vi "Main.vi"(11 "Module Admin":refnum<class "Delacor_lib_QMH_Cloneable Module Admin.lvclass">) -> ()   [LabVIEW 2020, in "FGen.lvlib"]
doc: "This template is based off of the Queued Message Handler design pattern and the Queued Message Handler project template that ships with LabVIEW.\n\nThe main difference is that the queue is private to this module and communication between modules is performed via Broadcast and Request events.\n\nRequest events are wrapped in public API methods and are handled in the Event Handling Loop (EHL) of this VI. Any module can register for Broadcast events sent by this module. The EHL generates messages based on user interface actions.\n\nThe Message Handling Loop (MHL) processes messages generated by the EHL, or by other messages. The messages are string values, so new messages can be added easily to the Message Cases case structure in the MHL. Each message cluster can also provide an optional value for Message Data, which is a variant that can be converted to whatever message-specific data is required.\n_____\nBased on DQMH Project Template 6.0.0.91."
uses:
  FGen.lvlib
  <vilib>/Delacor/Delacor QMH/Libraries/Cloneable Module Admin_class/Delacor_lib_QMH_Cloneable Module Admin.lvclass
  C:/Program Files (x86)/National Instruments/LabVIEW 2020/vi.lib/Delacor/Delacor QMH/Libraries/Module Admin_class/Delacor_lib_QMH_Module Admin.lvclass
  Module Data--cluster.ctl
  Generador/Generador.lvclass
  <vilib>/Delacor/Delacor QMH/Libraries/Message Queue_class/Delacor_lib_QMH_Message Queue.lvclass/Delacor_lib_QMH_Message Queue.ctl
  <vilib>/Delacor/Delacor QMH/Libraries/Cloneable Module Admin_class/Delacor_lib_QMH_Cloneable Module Admin.lvclass/Delacor_lib_QMH_Cloneable Module Admin.ctl
  Stop Argument--cluster.ctl
  <vilib>/Delacor/Delacor QMH/Libraries/Module Admin_class/Delacor_lib_QMH_Module Admin.lvclass/Delacor_lib_QMH_Module Admin.ctl
  Set Signal Type Argument--cluster.ctl
  Set to Default Argument--cluster.ctl
  Generate Signal Argument--cluster.ctl
  Generate Signal (Reply Payload)--cluster.ctl
  <vilib>/Utility/miscctls.llb/LVPointTypeDef.ctl
  Generador/Generador.lvclass/Generador.ctl
  <vilib>/Delacor/Delacor QMH/Libraries/Message Queue_class/Delacor_lib_QMH_Enqueue Message (Single).vi
  <vilib>/Delacor/Delacor QMH/Libraries/Cloneable Module Admin_class/Delacor_lib_QMH_Get Module ID.vi
  <vilib>/Delacor/Delacor QMH/Libraries/Module Admin_class/Delacor_lib_QMH_Get External Launch.vi
  <vilib>/Utility/error.llb/Error Cluster From Error Code.vi
  <vilib>/ErrorRing/Error Ring.xnode
  <vilib>/Delacor/Delacor QMH/Libraries/Message Queue_class/Delacor_lib_QMH_Message Queue.lvclass
panel:
  out "error out":errorcluster
  out "Status":string
  in  "Simulate EHL Error":bool
  in  "Simulate MHL Error":bool
  # "Other QMH Modules communicate with this Module via its Public API (wrappers for its Request Events).\n\nThis Module communicates with other Modules via its Broadcast Events.\nAny module that wants to get these messages, just registers for this module's Broadcast events."
  # "This template is for the Delacor Modified Queued Message Handler design pattern.\n\nSee the block diagram for more information on how to use this template."
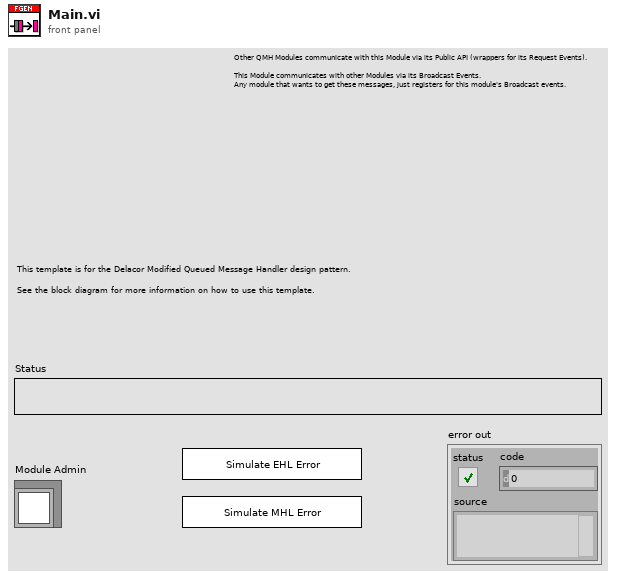
[diagram p1: front panel]
types:
  T1 = typedef "FGen.lvlib/Request Events--cluster.ctl" = cluster{"Stop Module":refnum<user-event>, "Show Panel":refnum<user-event>, "Hide Panel":refnum<user-event>, "Show Diagram":refnum<user-event>, "Get Module Execution Status":refnum<user-event>, "Set Signal Type":refnum<user-event>, "Set to Default":refnum<user-event>, "Generate Signal":refnum<user-event>}
  T2 = typedef "FGen.lvlib/Module Data--cluster.ctl" = cluster{"Status":string, "Generator":refnum<class "Generador.lvclass">}
  T3 = enum32{"invalid lock state", "Not Locked", "Locked (No Password)", "Password-protected"}
  T4 = typedef "FGen.lvlib/Stop Argument--cluster.ctl" = cluster{"Module ID":i32, "Origin":string, "Exit via Stop Module Req?":bool, "Wait for Module to stop?":bool}
  T5 = typedef "FGen.lvlib/Set Signal Type Argument--cluster.ctl" = cluster{"Module ID":i32, "signal type":enum16{"Sine Wave", "Triangle Wave", "Square Wave", "Sawtooth Wave"}}
  T6 = typedef "FGen.lvlib/Set to Default Argument--cluster.ctl" = cluster{"Module ID":i32, "Boolean":bool}
  T7 = typedef "FGen.lvlib/Generate Signal Argument--cluster.ctl" = cluster{"Module ID":i32, "Wait Notifier":refnum<notifier>, "wait for reply":bool}
  T8 = typedef "LVPointTypeDef.ctl" = cluster{"Horizontal":i16, "Vertical":i16}
  T9 = enum32{"Invalid", "Standard", "Closed", "Hidden", "Minimized", "Maximized"}
  T10 = typedef "FGen.lvlib/Generate Signal (Reply Payload)--cluster.ctl" = cluster{"signal out":waveform(dbl), "Generate Signal_error":errorcluster}
  T11 = enum16{"Sine Wave", "Triangle Wave", "Square Wave", "Sawtooth Wave"}
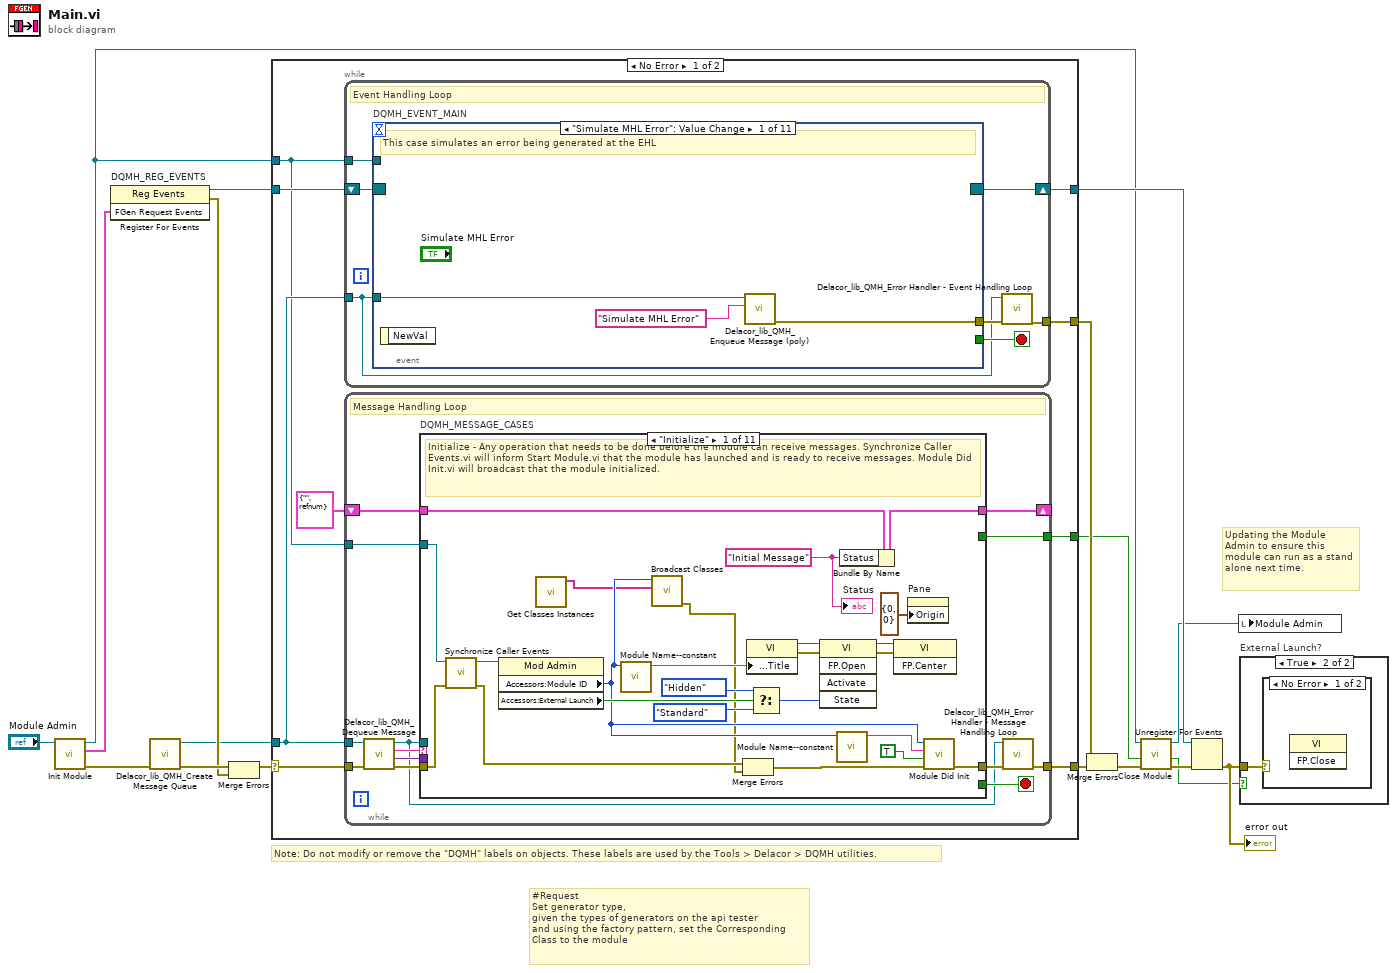
[diagram p0: block diagram]
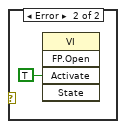
[diagram p3: hidden frame]
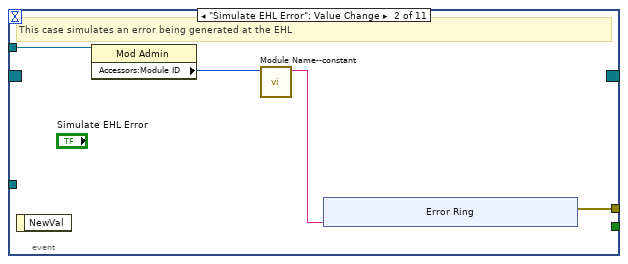
[diagram p4: hidden frame]
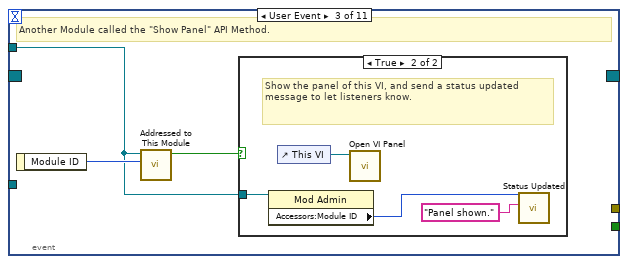
[diagram p5: hidden frame]
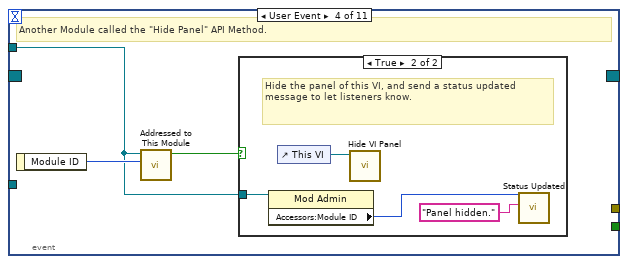
[diagram p7: hidden frame]
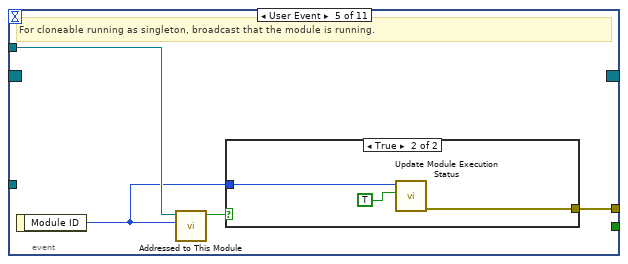
[diagram p9: hidden frame]
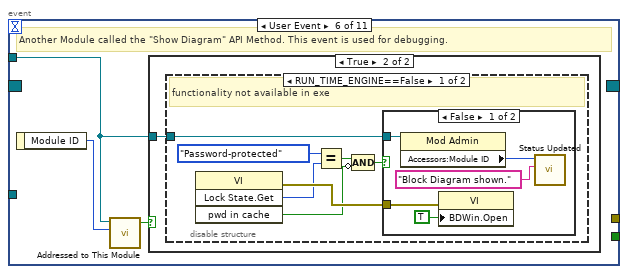
[diagram p11: hidden frame]
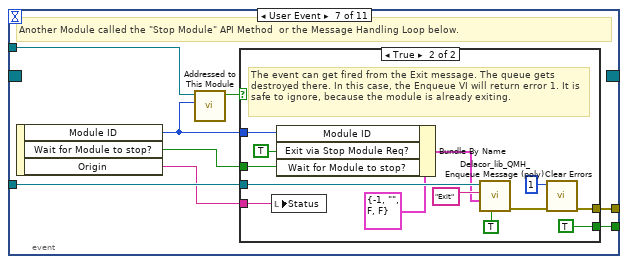
[diagram p15: hidden frame]
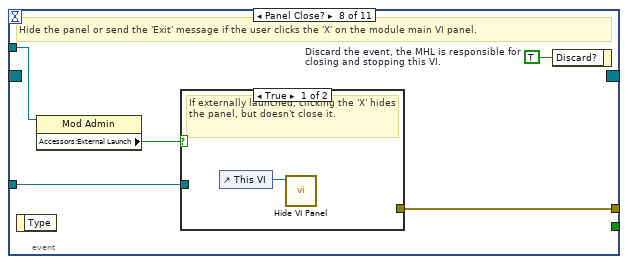
[diagram p17: hidden frame]
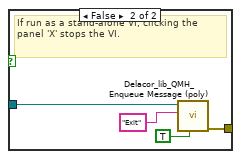
[diagram p18: hidden frame]
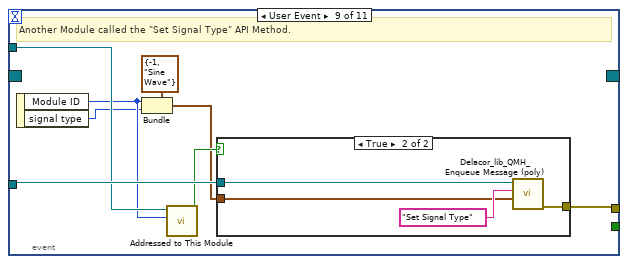
[diagram p19: hidden frame]
diagram:
  # "#Request\nSet generator type, \ngiven the types of generators on the api tester\nand using the factory pattern, set the Corresponding\nClass to the module"
  # "Note: Do not modify or remove the \"DQMH\" labels on objects. These labels are used by the Tools > Delacor > DQMH utilities."
  # "Updating the Module Admin to ensure this module can run as a stand alone next time."
  n1 = call "Init Module.vi"("Cloneable Module Admin in"="Module Admin") -> ("error out"=w15:errorcluster, "FGen Request Events"=w7:T1, "Cloneable Module Admin out"=w4:refnum<class "Delacor_lib_QMH_Cloneable Module Admin.lvclass">)  [unwired: 8 in]
  n2 = register-events "DQMH_REG_EVENTS"(w7) -> (reference out=w8:refnum<event-registration>, error out=w10:errorcluster)  [unwired: 2 in]
  n3 = call <vilib>:"Delacor_lib_QMH_Create Message Queue.vi"("error in"=w15) -> ("error out"=w12:errorcluster, "Message Queue"=w6:refnum<class "Delacor_lib_QMH_Message Queue.lvclass">)  [unwired: 9 in]
  n4 = Merge Errors(w12, w10) -> (w11:errorcluster)
  n5 = case shown="No Error" w11 {
    selector: w11 -> [w25 w304]
    tunnel: [w27 w303] -> w16
    tunnel: [w24 w311] -> w9
    tunnel: w8 -> [w22 w311]
    tunnel: w6 -> [w21 w302]
    tunnel: [w26 _] -> w17
    tunnel: w4 -> [w20 w307]
    tunnel: [w19 _] -> w2
    frame No Error {
      n6 = while {
        tunnel: w21 -> [w28]
        shift-right: [w31] -> w24
        shift-left: w22 -> [w32]
        tunnel: [w33] -> w26
        tunnel: w20 -> [w29]
        stop <- w30 stop-if-true
        # "Event Handling Loop"
        n7 = event "DQMH_EVENT_MAIN" shown="[0] \"Simulate MHL Error\": Value Change" {
          selector: w32 -> [_ _ _ _ _ _ _ _ _ _ _]
          dyn-events: [_ _ _ _ _ _ _ _ _ _ _] -> w31
          timeout: _ -> [_ _ _ _ _ _ _ _ _ _ _]
          tunnel: [_ _ _ _ _ _ w89 _ _ _ _] -> w30
          tunnel: w28 -> [w36 _ _ _ _ _ w92 w108 w124 w136 w149]
          tunnel: [w37 w41 _ _ w66 _ w93 w111 w117 w129 w141] -> w34
          tunnel: w29 -> [_ w40 w49 w56 w64 w70 w91 w109 w122 w134 w147]
          event "Simulate MHL Error": Value Change {
            # "This case simulates an error being generated at the EHL"
            n8 = event-data() -> ()  [unwired: 1 in, 1 out]
            n9 = call-poly <vilib>:"Delacor_lib_QMH_Enqueue Message (poly).vi"("Message"="Simulate MHL Error", "Message Queue in"=w36) -> ("error out"=w37:errorcluster)  [unwired: 8 in, 1 out]
          }
          event "Simulate EHL Error": Value Change {
            # "This case simulates an error being generated at the EHL"
            n10 = event-data() -> ()  [unwired: 1 in, 1 out]
            n11 = property class="Mod Admin"(reference=w40) -> ("Accessors:Module ID"=w39:i32)  [unwired: 1 in, 2 out]
            n12 = call "Module Name--constant.vi"("Module ID"=w39) -> ("Module Name"=w38:string)  [unwired: 10 in]
            n13 = xnode "Error Ring"("parameter 0"=w38) -> ("error out"=w41:errorcluster)
          }
          event User Event {
            # "Another Module called the \"Show Panel\" API Method."
            n14 = event-data() -> ("Module ID"=w50:i32)  [unwired: 1 in]
            n15 = call "Addressed to This Module.vi"("Module ID from Argument"=w50, "Module Admin"=w49) -> ("Addressed to this instance?"=w51:bool)  [unwired: 8 in, 1 out]
            n16 = case shown="True" w51 {
              tunnel: w49 -> [_ w53]
              frame False {
              }
              frame True {
                # "Show the panel of this VI, and send a status updated message to let listeners know."
                n17 = property class="Mod Admin"(reference=w53) -> ("Accessors:Module ID"=w52:i32)  [unwired: 1 in, 2 out]
                n18 = control-ref of="This VI"() -> (w55:refnum<vi>)
                n19 = call "Open VI Panel.vi"("VI"=w55) -> ()  [unwired: 10 in, 1 out]
                n20 = call "Status Updated.vi"("Status"="Panel shown." ("format string"), "Module ID"=w52) -> ()  [unwired: 9 in, 1 out]
              }
            }
          }
          event User Event {
            # "Another Module called the \"Hide Panel\" API Method."
            n21 = event-data() -> ("Module ID"=w57:i32)  [unwired: 1 in]
            n22 = call "Addressed to This Module.vi"("Module ID from Argument"=w57, "Module Admin"=w56) -> ("Addressed to this instance?"=w58:bool)  [unwired: 8 in, 1 out]
            n23 = case shown="True" w58 {
              tunnel: w56 -> [_ w60]
              frame False {
              }
              frame True {
                # "Hide the panel of this VI, and send a status updated message to let listeners know."
                n24 = property class="Mod Admin"(reference=w60) -> ("Accessors:Module ID"=w59:i32)  [unwired: 1 in, 2 out]
                n25 = control-ref of="This VI"() -> (w62:refnum<vi>)
                n26 = call "Hide VI Panel.vi"("VI"=w62) -> ()  [unwired: 10 in, 1 out]
                n27 = call "Status Updated.vi"("Status"="Panel hidden." ("format string"), "Module ID"=w59) -> ()  [unwired: 9 in, 1 out]
              }
            }
          }
          event User Event {
            # "For cloneable running as singleton, broadcast that the module is running."
            n28 = event-data() -> ("Module ID"=w63:i32)  [unwired: 1 in]
            n29 = call "Addressed to This Module.vi"("Module ID from Argument"=w63, "Module Admin"=w64) -> ("Addressed to this instance?"=w65:bool)  [unwired: 8 in, 1 out]
            n30 = case shown="True" w65 {
              tunnel: [_ w69] -> w66
              tunnel: w63 -> [_ w68]
              frame False {
              }
              frame True {
                n31 = call "Update Module Execution Status.vi"("Running?"=TRUE, "Module ID"=w68) -> ("error out"=w69:errorcluster)  [unwired: 9 in]
              }
            }
          }
          event User Event {
            # "Another Module called the \"Show Diagram\" API Method. This event is used for debugging."
            n32 = event-data() -> ("Module ID"=w71:i32)  [unwired: 1 in]
            n33 = call "Addressed to This Module.vi"("Module ID from Argument"=w71, "Module Admin"=w70) -> ("Addressed to this instance?"=w72:bool)  [unwired: 8 in, 1 out]
            n34 = case shown="True" w72 {
              tunnel: w70 -> [_ w73]
              frame False {
              }
              frame True {
                n35 = disable-structure shown="RUN_TIME_ENGINE==False" {
                  disable-tunnel: w73 -> [w74 _]
                  frame condition #0 (active) {
                    # "functionality not available in exe"
                    n36 = invoke class="VI" method="Lock State.Get"() -> (error out=w80:errorcluster, "Get Lock State"=w79:T3, "pwd in cache"=w76:bool)  [unwired: 4 in, 1 out]
                    n37 = Equal?(x=T3."Password-protected", y=w79) -> (x = y?=w77:bool)
                    n38 = Compound Arithmetic op=AND(w77, invert w76) -> (w75:bool)
                    n39 = case shown="False" w75 {
                      tunnel: w80 -> [w85 _]
                      tunnel: w74 -> [w82 _]
                      frame False {
                        n40 = property class="Mod Admin"(reference=w82) -> ("Accessors:Module ID"=w81:i32)  [unwired: 1 in, 2 out]
                        n41 = property class="VI"(error in=w85, "BDWin.Open"=TRUE ("Block Diagram Window:Open")) -> ()  [unwired: 1 in, 2 out]
                        n42 = call "Status Updated.vi"("Status"="Block Diagram shown." ("format string"), "Module ID"=w81) -> ()  [unwired: 9 in, 1 out]
                      }
                      frame True {
                        # "Password-protected VI, and the password is not in the cache. Do not show the diagram."
                      }
                    }
                  }
                  frame condition #1 {
                  }
                }
              }
            }
          }
          event User Event {
            # "Another Module called the \"Stop Module\" API Method  or the Message Handling Loop below."
            n43 = event-data() -> ("Module ID"=w87:i32, "Wait for Module to stop?"=w88:bool, "Origin"=w86:string)  [unwired: 1 in]
            n44 = call "Addressed to This Module.vi"("Module ID from Argument"=w87, "Module Admin"=w91) -> ("Addressed to this instance?"=w90:bool)  [unwired: 8 in, 1 out]
            n45 = case shown="True" w90 {
              tunnel: [_ w105] -> w93
              tunnel: w92 -> [_ w101]
              tunnel: [_ TRUE] -> w89
              tunnel: w88 -> [_ w96]
              tunnel: w87 -> [_ w98]
              tunnel: w86 -> [_ w94]
              frame False {
              }
              frame True {
                # "The event can get fired from the Exit message. The queue gets destroyed there. In this case, the Enqueue VI will return error 1. It is safe to ignore, because the module is already exiting."
                n46 = local write "Status"(w94) -> ()
                n47 = Bundle By Name(cluster=T4 {"Module ID"=-1, "Origin"="", "Exit via Stop Module Req?"=FALSE, "Wait for Module to stop?"=FALSE} ("Stop Argument"), "Module ID"=w98, "Exit via Stop Module Req?"=TRUE, "Wait for Module to stop?"=w96) -> (w95:T4)
                n48 = call-poly <vilib>:"Delacor_lib_QMH_Enqueue Message (poly).vi"("Priority Message? (F)"=TRUE, "Message Data"=w95, "Message"="Exit", "Message Queue in"=w101) -> ("error out"=w106:errorcluster)  [unwired: 6 in, 1 out]
                n49 = call <vilib>:"Clear Errors.vi"("error in (no error)"=w106, "specific error code to clear (0: all)"=1) -> ("error out"=w105:errorcluster)  [unwired: 4 in, 1 out]
              }
            }
          }
          event Panel Close? {
            w110 = TRUE  # Discard the event, the MHL is responsible for closing and stopping this VI.
            # "Hide the panel or send the 'Exit' message if the user clicks the 'X' on the module main VI panel."
            n50 = event-data() -> ()  [unwired: 1 in, 1 out]
            n51 = property class="Mod Admin"(reference=w109) -> ("Accessors:External Launch"=w107:bool)  [unwired: 1 in, 2 out]
            n52 = case shown="True" w107 {
              tunnel: w108 -> [_ w115]
              tunnel: [_ w116] -> w111
              frame True {
                # "If externally launched, clicking the 'X' hides the panel, but doesn't close it."
                n53 = control-ref of="This VI"() -> (w112:refnum<vi>)
                n54 = call "Hide VI Panel.vi"("VI"=w112) -> ()  [unwired: 10 in, 1 out]
              }
              frame False {
                # "If run as a stand-alone VI, clicking the panel 'X' stops the VI."
                n55 = call-poly <vilib>:"Delacor_lib_QMH_Enqueue Message (poly).vi"("Priority Message? (F)"=TRUE, "Message"="Exit", "Message Queue in"=w115) -> ("error out"=w116:errorcluster)  [unwired: 7 in, 1 out]
              }
            }
            n56 = event-data("Discard?"=w110) -> ()  [unwired: 1 in, 1 out]
          }
          event User Event {
            # "Another Module called the \"Set Signal Type\" API Method."
            n57 = event-data() -> ("Module ID"=w119:i32, "signal type"=w118:T11)  [unwired: 1 in]
            n58 = Bundle(cluster=T5 {"Module ID"=-1, "signal type"=enum."Sine Wave"} ("Set Signal Type Argument"), "Module ID"=w119, "signal type"=w118) -> (w120:T5)
            n59 = call "Addressed to This Module.vi"("Module ID from Argument"=w119, "Module Admin"=w122) -> ("Addressed to this instance?"=w123:bool)  [unwired: 8 in, 1 out]
            n60 = case shown="True" w123 {
              tunnel: w124 -> [_ w128]
              tunnel: w120 -> [_ w126]
              tunnel: [_ w125] -> w117
              frame False {
              }
              frame True {
                n61 = call-poly <vilib>:"Delacor_lib_QMH_Enqueue Message (poly).vi"("Message Data"=w126, "Message"="Set Signal Type", "Message Queue in"=w128) -> ("error out"=w125:errorcluster)  [unwired: 7 in, 1 out]
              }
            }
          }
          event User Event {
            # "Another Module called the \"Set to Default\" API Method."
            n62 = event-data() -> ("Module ID"=w131:i32, "Boolean"=w130:bool)  [unwired: 1 in]
            n63 = Bundle(cluster=T6 {"Module ID"=-1, "Boolean"=FALSE} ("Set to Default Argument"), "Module ID"=w131, "Boolean"=w130) -> (w132:T6)
            n64 = call "Addressed to This Module.vi"("Module ID from Argument"=w131, "Module Admin"=w134) -> ("Addressed to this instance?"=w135:bool)  [unwired: 8 in, 1 out]
            n65 = case shown="True" w135 {
              tunnel: w136 -> [_ w140]
              tunnel: w132 -> [_ w138]
              tunnel: [_ w137] -> w129
              frame False {
              }
              frame True {
                n66 = call-poly <vilib>:"Delacor_lib_QMH_Enqueue Message (poly).vi"("Message Data"=w138, "Message"="Set to Default", "Message Queue in"=w140) -> ("error out"=w137:errorcluster)  [unwired: 7 in, 1 out]
              }
            }
          }
          event User Event {
            # "Another Module called the \"Generate Signal\" API Method."
            n67 = event-data() -> ("Module ID"=w144:i32, "Wait Notifier"=w143:refnum<notifier>, "wait for reply"=w142:bool)  [unwired: 1 in]
            n68 = Bundle(cluster=T7 {"Module ID"=-1, "Wait Notifier"=refnum, "wait for reply"=FALSE} ("Generate Signal Argument"), "Module ID"=w144, "Wait Notifier"=w143, "wait for reply"=w142) -> (w145:T7)
            n69 = call "Addressed to This Module.vi"("Module ID from Argument"=w144, "Module Admin"=w147) -> ("Addressed to this instance?"=w148:bool)  [unwired: 8 in, 1 out]
            n70 = case shown="True" w148 {
              tunnel: w149 -> [_ w153]
              tunnel: w145 -> [_ w151]
              tunnel: [_ w150] -> w141
              frame False {
              }
              frame True {
                n71 = call-poly <vilib>:"Delacor_lib_QMH_Enqueue Message (poly).vi"("Message Data"=w151, "Message"="Generate Signal", "Message Queue in"=w153) -> ("error out"=w150:errorcluster)  [unwired: 7 in, 1 out]
              }
            }
          }
        }
        n72 = call-dynamic "Delacor_lib_QMH_Error Handler - Event Handling Loop.vi"("error in"=w34, "Message Queue in"=w28) -> ("dup error in"=w33:errorcluster)  [unwired: 8 in, 1 out]
      }
      n73 = while {
        tunnel: w21 -> [w157]
        shift-right: [w161] -> _
        shift-left: T2 {"Status"="", "Generator"=refnum} ("Data Cluster") -> [w162]
        tunnel: w25 -> [w165]
        tunnel: [w163] -> w27
        tunnel: w20 -> [w155]
        tunnel: [w154] -> w19
        stop <- w160 stop-if-true
        # "Message Handling Loop"
        n74 = call-dynamic "Delacor_lib_QMH_Dequeue Message.vi"("error in"=w165, "Message Queue in"=w157) -> ("error out"=w164:errorcluster, "Message Data"=w158:variant, "Message"=w159:string, "Message Queue out"=w156:refnum<class "Delacor_lib_QMH_Message Queue.lvclass">)  [unwired: 6 in]
        n75 = case "DQMH_MESSAGE_CASES" shown="\"Initialize\"" w159 {
          selector: w159 -> [_ _ _ _ _ _ _ _ _ _ w289]
          tunnel: w156 -> [_ _ _ _ _ _ _ w240 _ w279 _]
          tunnel: w164 -> [w188 w192 w202 w212 w230 w236 w238 w249 w262 w285 w291]
          tunnel: [w186 w192 w201 w211 w221 w235 w238 w245 w261 w282 w292] -> w166
          tunnel: w162 -> [w179 w191 w195 w206 w215 w234 w237 w244 w259 w278 w290]
          tunnel: [w178 w191 w194 w205 w214 w234 w237 w244 w259 w278 w290] -> w161
          tunnel: [_ _ _ _ _ _ _ _ _ w277 _] -> w160
          tunnel: w158 -> [_ _ w200 w210 w228 _ _ w243 _ w275 _]
          tunnel: w155 -> [w174 _ _ _ _ _ _ w242 w257 w271 w287]
          tunnel: [_ _ _ _ _ _ _ _ _ w273 _] -> w154
          frame "Initialize" {
            w171 = "Initial Message" ("Initial Message")
            # "Initialize - Any operation that needs to be done before the module can receive messages. Synchronize Caller Events.vi will inform Start Module.vi that the module has launched and is ready to receive messages. Module Did Init.vi will broadcast that the module initialized."
            n76 = call "Synchronize Caller Events.vi"("error in (no error)"=w188, "Module Admin"=w174) -> ("error out"=w187:errorcluster, "Module Admin out"=w173:refnum<class "Delacor_lib_QMH_Cloneable Module Admin.lvclass">)  [unwired: 8 in]
            n77 = property class="Mod Admin"(reference=w173) -> ("Accessors:Module ID"=w170:i32, "Accessors:External Launch"=w175:bool)  [unwired: 1 in, 2 out]
            n78 = call "Get Classes Instances.vi"() -> ("Classes"=w169:string[])  [unwired: 11 in]
            n79 = call "Module Name--constant.vi"("Module ID"=w170) -> ("Module Name"=w183:string)  [unwired: 10 in]
            n80 = call "Broadcast Classes.vi"("Classes"=w169, "Module ID"=w170) -> ("error out"=w167:errorcluster)  [unwired: 9 in]
            n81 = Merge Errors(w187, w167) -> (w168:errorcluster)
            n82 = property class="VI"("Front Panel.Title"=w183) -> (reference out=w185:refnum<vi>, error out=w190:errorcluster)  [unwired: 2 in]
            n83 = Select(t=T9."Hidden" ("State"), s=w175, f=T9."Standard" ("State")) -> (s? t:f=w180:T9)
            n84 = invoke class="VI" method="FP.Open"(reference=w185, error in=w190, "State"=w180) -> (reference out=w184:refnum<vi>, error out=w189:errorcluster)  [unwired: 2 in, 3 out]
            n85 = call "Module Name--constant.vi"("Module ID"=w170) -> ("Module Name"=w176:string)  [unwired: 10 in]
            n86 = Bundle By Name(cluster=w179, "Status"=w171) -> (w178:T2)
            n87 = invoke class="VI" method="FP.Center"(reference=w184, error in=w189) -> ()  [unwired: 1 in, 3 out]
            n88 = property on="Pane" class="Pane"("Origin"=T8 {"Horizontal"=0, "Vertical"=0}) -> ()  [unwired: 2 in, 2 out]
            n89 = call "Module Did Init.vi"("error in (no error)"=w168, "Initialized?"=TRUE, "Origin"=w176, "Module ID"=w170) -> ("error out"=w186:errorcluster)  [unwired: 7 in]
            "Status" <- w171
          }
          frame "---Module Specific---" {
            # "Separator -- The following cases handle messages specific to this Module."
          }
          frame "Set Signal Type" {
            # "#CompleteMissingCode\nAdd the output Object of the method to the Module Data"
            # "Set the Signal type to be generated"
            n90 = Variant To Data(error in=w202, type=T5 {"Module ID"=-1, "signal type"=enum."Sine Wave"} ("Set Signal Type Argument"), Variant=w200) -> (data=w198:T5, error out=w201:errorcluster)
            n91 = Unbundle By Name(w198) -> ("signal type"=w196:T11)
            n92 = Unbundle By Name(w195) -> ("Generator"=w197:refnum<class "Generador.lvclass">)
            n93 = call "Set signal type.vi"("signal type"=w196, "Generator in"=w197) -> ("Generator out"=w193:refnum<class "Generador.lvclass">)  [unwired: 8 in, 1 out]
            n94 = in-place {
              in-place-border: w193 -> [w203]
              n95 = in-place-cluster #1(w195) -> ()  [unwired: 1 out]
              n96 = in-place-cluster #1("Generator"=w203) -> (w194:T2)
            }
          }
          frame "Set to Default" {
            # "#CompleteMissingCode\nAdd the output Object of the method to the Module Data"
            # "Set the signal to default values"
            n97 = Variant To Data(error in=w212, type=T6 {"Module ID"=-1, "Boolean"=FALSE} ("Set to Default Argument"), Variant=w210) -> (data=w208:T6, error out=w211:errorcluster)
            n98 = Unbundle By Name(w206) -> ("Generator"=w207:refnum<class "Generador.lvclass">)
            n99 = Unbundle By Name(w208) -> ()  [unwired: 2 out]
            n100 = call-dynamic "Default--constant.vi"("Generator in"=w207) -> ("Generator out"=w204:refnum<class "Generador.lvclass">)  [unwired: 9 in, 1 out]
            n101 = in-place {
              in-place-border: w204 -> [w213]
              n102 = in-place-cluster #2(w206) -> ()  [unwired: 1 out]
              n103 = in-place-cluster #2("Generator"=w213) -> (w205:T2)
            }
          }
          frame "Generate Signal" {
            # "#CompleteMissingCode\nAdd the class to the method"
            # "Generate the signal with the Defined values"
            n104 = Unbundle By Name(w215) -> ("Generator"=w219:refnum<class "Generador.lvclass">)
            n105 = Variant To Data(error in=w230, type=T7 {"Module ID"=-1, "Wait Notifier"=refnum, "wait for reply"=FALSE} ("Generate Signal Argument"), Variant=w228) -> (data=w226:T7, error out=w229:errorcluster)
            n106 = Unbundle By Name(w226) -> ("Wait Notifier"=w225:refnum<notifier>, "wait for reply"=w224:bool)  [unwired: 1 out]
            n107 = call "Generate Waveform.vi"("Generator in"=w219) -> ("error out"=w218:errorcluster, "Waveform"=w220:waveform(dbl), "Generator out"=w216:refnum<class "Generador.lvclass">)  [unwired: 8 in]
            n108 = Bundle By Name(cluster=w215, "Generator"=w216) -> (w214:T2)
            n109 = Bundle By Name(cluster=T10 {"signal out"={"t0"=timestamp(0 s since 1904-01-01), "dt"=1.0, "Y"=[]}, "Generate Signal_error"={"status"=FALSE, "code"=0, "source"=""}} ("Generate Signal (Reply Payload)"), "signal out"=w220, "Generate Signal_error"=w218) -> (w223:T10)
            n110 = case shown="True" w224 {
              tunnel: w225 -> [_ w233]
              tunnel: w223 -> [_ w232]
              tunnel: [_ w231] -> w217
              frame False {
              }
              frame True {
                n111 = Send Notification(notification=w232, notifier=w233) -> (error out=w231:errorcluster)  [unwired: 1 in, 1 out]
              }
            }
            n112 = Merge Errors(w229, w217) -> (w221:errorcluster)
          }
          frame "---Copy This Frame---" {
            # "Duplicate this frame when creating new messages.  Change this comment in the duplicated frame to describe this message."
            n113 = Merge Errors(w236) -> (w235:errorcluster)
          }
          frame "---Exit and Error Handling---" {
            # "Separator - the following cases handle errors and exit messages."
          }
          frame "Error" {
            # "Error - Check the error message data and respond accordingly. This message is sent by the \"Error Handler\" VIs at the end of each loop in this application."
            n114 = property class="Mod Admin"(reference=w242) -> ("Accessors:External Launch"=w241:bool, "Accessors:Module ID"=w239:i32)  [unwired: 1 in, 2 out]
            n115 = Variant To Data(error in=w249, type=errorcluster {"status"=FALSE, "code"=0, "source"=""} ("error constant"), Variant=w243) -> (data=w250:errorcluster, error out=w247:errorcluster)
            n116 = call "Error Reported.vi"("Error"=w250, "Module ID"=w239) -> ()  [unwired: 9 in, 1 out]
            n117 = case shown="False" w241 {
              tunnel: [w255 _] -> w246
              tunnel: w240 -> [w253 _]
              tunnel: w250 -> [w254 _]
              frame False {
                # "If the module is running standalone, then pop up an error dialog and call the \"Exit\" message."
                n118 = call <vilib>:"Simple Error Handler.vi"("error in (no error)"=w254) -> ()  [unwired: 4 in, 5 out]
                n119 = call-poly <vilib>:"Delacor_lib_QMH_Enqueue Message (poly).vi"("Priority Message? (F)"=TRUE, "Message"="Exit", "Message Queue in"=w253) -> ("error out"=w255:errorcluster)  [unwired: 7 in, 1 out]
              }
              frame True {
                # "If the module was launched externally, calling the Error Reported broadcast VI is the only action performed by the \"Error\" message. The module's caller can then process the error appropriately."
              }
            }
            n120 = Merge Errors(w247, w246) -> (w245:errorcluster)
            n121 = local write "error out"(w245) -> ()
          }
          frame "Simulate MHL Error" {
            # "Simulate an error occurring at the MHL"
            n122 = property class="Mod Admin"(reference=w257) -> ("Accessors:Module ID"=w258:i32)  [unwired: 1 in, 2 out]
            n123 = call "Module Name--constant.vi"("Module ID"=w258) -> ("Module Name"=w256:string)  [unwired: 10 in]
            n124 = xnode "Error Ring"("parameter 0"=w256) -> ("error out"=w260:errorcluster)
            n125 = Merge Errors(w262, w260) -> (w261:errorcluster)
          }
          frame "Exit" {
            w276 = 91  # 91: not all Exit messages will have an argument
            w277 = TRUE  # Stop the VI
            # "Release the message queue reference"
            # "Exit - Exit the application."
            n126 = Variant To Data(error in=w285, type=T4 {"Module ID"=-1, "Origin"="", "Exit via Stop Module Req?"=FALSE, "Wait for Module to stop?"=FALSE} ("Stop Argument"), Variant=w275) -> (data=w272:T4, error out=w280:errorcluster)
            n127 = call <vilib>:"Clear Errors.vi"("error in (no error)"=w280, "specific error code to clear (0: all)"=w276) -> ("error out"=w284:errorcluster)  [unwired: 4 in, 1 out]
            n128 = control-ref of="This VI"() -> (w270:refnum<vi>)
            n129 = call-dynamic "Delacor_lib_QMH_Release Message Queue.vi"("error in"=w284, "Message Queue"=w279) -> ("error out"=w283:errorcluster)  [unwired: 9 in]
            n130 = call "Handle Exit.vi"("Stop Argument"=w272, "Module Admin in"=w271, "VI reference"=w270) -> ("error out"=w281:errorcluster, "Wait for Stop?"=w273:bool)  [unwired: 7 in]
            n131 = Merge Errors(w283, w281) -> (w282:errorcluster)
          }
          frame Default {
            # "'Default' case only runs if there is a message that isn't defined in any of the other cases.  Output a programming error."
            n132 = property class="Mod Admin"(reference=w287) -> ("Accessors:Module ID"=w286:i32)  [unwired: 1 in, 2 out]
            n133 = call "Module Name--constant.vi"("Module ID"=w286) -> ("Module Name"=w288:string)  [unwired: 10 in]
            n134 = xnode "Error Ring"("parameter 0"=w289, "parameter 1"=w288) -> ("error out"=w293:errorcluster)
            n135 = Merge Errors(w291, w293) -> (w292:errorcluster)
          }
        }
        n136 = call-dynamic "Delacor_lib_QMH_Error Handler - Message Handling Loop.vi"("error in"=w166, "Message Queue in"=w156) -> ("dup error in"=w163:errorcluster)  [unwired: 8 in, 1 out]
      }
    }
    frame Error {
      n137 = call "Synchronize Caller Events.vi"("Module Admin"=w307) -> ("Module Admin out"=w306:refnum<class "Delacor_lib_QMH_Cloneable Module Admin.lvclass">)  [unwired: 9 in, 1 out]
      n138 = property class="Mod Admin"(reference=w306) -> ("Accessors:Module ID"=w305:i32)  [unwired: 1 in, 2 out]
      n139 = call-dynamic "Delacor_lib_QMH_Release Message Queue.vi"("error in"=w304, "Message Queue"=w302) -> ("error out"=w303:errorcluster)  [unwired: 9 in]
      n140 = call "Module Name--constant.vi"("Module ID"=w305) -> ("Module Name"=w310:string)  [unwired: 10 in]
      n141 = Format Into String(format string="An error occurred during initialization. %s is no longer running.", w310) -> (resulting string=w308:string)  [unwired: 2 in, 1 out]
      n142 = call "Error Reported.vi"("Additional Information"=w308, "Error"=w303, "Module ID"=w305) -> ()  [unwired: 8 in, 1 out]
    }
  }
  n143 = Merge Errors(w17, w16) -> (w18:errorcluster)
  n144 = call "Close Module.vi"("error in"=w18, "Wait for stop?"=w2, "Module Admin in"=w4) -> ("error out"=w14:errorcluster, "External Launch"=w1:bool, "Module Admin out"=w3:refnum<class "Delacor_lib_QMH_Cloneable Module Admin.lvclass">)  [unwired: 6 in]
  n145 = Unregister For Events(event registration refnum=w9, error in=w14) -> (error out=w13:errorcluster)
  "error out" <- w13
  n146 = local write "Module Admin"(w3) -> ()
  n147 = case "External Launch?" shown="True" w1 {
    tunnel: w13 -> [_ w312]
    frame False {
    }
    frame True {
      n148 = case shown="No Error" w312 {
        frame No Error {
          n149 = invoke class="VI" method="FP.Close"() -> ()  [unwired: 3 in, 3 out]
        }
        frame Error {
          n150 = invoke class="VI" method="FP.Open"("Activate"=TRUE ("Activate?")) -> ()  [unwired: 4 in, 5 out]
        }
      }
    }
  }
